vi "Detect Collision with HAB.vi"(1 "Right Current":dbl, 2 "Right Velocity":dbl, 3 "Left Current":dbl, 4 "Left Velocity":dbl) -> (0 "HIT WALL":bool)   [LabVIEW 2018]
panel:
  in  "Current Threshold":dbl=6.5
  in  "Velocity Threshold":dbl=20.0
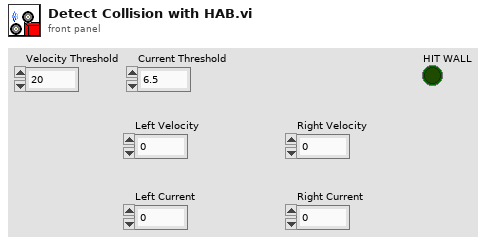
[diagram p1: front panel]
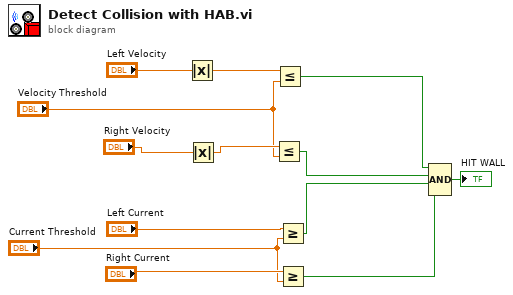
[diagram p0: block diagram]
diagram:
  n1 = Absolute Value(x="Left Velocity") -> (abs(x)=w3:dbl)
  n2 = Absolute Value(x="Right Velocity") -> (abs(x)=w5:dbl)
  n3 = Less Or Equal?(x=w5, y="Velocity Threshold") -> (x <= y?=w10:bool)
  n4 = Less Or Equal?(x=w3, y="Velocity Threshold") -> (x <= y?=w11:bool)
  n5 = Greater Or Equal?(x="Left Current", y="Current Threshold") -> (x >= y?=w9:bool)
  n6 = Greater Or Equal?(x="Right Current", y="Current Threshold") -> (x >= y?=w8:bool)
  n7 = Compound Arithmetic op=AND(w11, w10, w9, w8) -> (→"HIT WALL":bool)
